vi "ISEG_HVBoard.constructor.vi"(0 "name":string, 2 "data in":string, 5 "error in (no error)":errorcluster) -> (14 "i ref out":refnum<vi>, 16 "data out":string, 19 "error out":errorcluster)   [LabVIEW 2014, in "ISEG_HVBoard.lvlib"]
doc: "This is the constructor of a class.\n\nLicense Agreement for this software:\n\nCopyright (C)\nGesellschaft für Schwerionenforschung, GSI\nPlanckstr. 1\n64291 Darmstadt\nGermany\n\nContact: D.Beck@gsi.de \n\nThis program is free software; you can redistribute it and/or modify it under the terms of the \nGNU General Public License as published by the Free Software Foundation; either version 2 of \nthe license, or (at your option) any later version.\n\nThis program is distributed in the hope that it will be useful, but WITHOUT ANY WARRANTY; \nwithout even the implied warranty of MERCHANTABILITY or FITNESS FOR A PARTICULAR PURPOSE. See the GNU General License for more details (http://www.gnu.org).\n\nGesellschaft für Schwerionenforschung, GSI\nPlanckstr. 1, 64291 Darmstadt, Germany\nFor all questions and ideas contact: M.Richter@gsi.de, H.Brand@gsi.de or D.Beck@gsi.de.\nLast update: 16-JUN-2004"
uses:
  ISEG_HVBoard.lvlib
  ISEG_HVBoard.i attribute.ctl
  ISEG_HVBoard.DIM Status.ctl
  CSCore/CSApplicationBaseClasses/DeviceBase/DeviceBase.myEventNames.ctl
  CSCore/CSApplicationBaseClasses/DeviceBase/DeviceBase.lvlib
  CSCore/CSSystem/CSSystemLib/CSSystemLib.lvlib
  CSCore/BaseProcess/BaseProcess.lvlib
panel:
  in  "CLASS.i attribute":T1 {"Status"."Status" format="%.0b"}
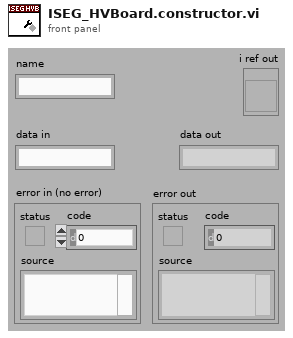
[diagram p1: front panel]
types:
  T1 = typedef "ISEG_HVBoard.lvlib/ISEG_HVBoard.i attribute.ctl" = cluster{"System Name":string, "Board ID":i32, "Prefix":string, "NrOfCh":cluster{"NrOfCh":i16, "DIM Status":T2}, "Status":cluster{"Status":i16, "DIM Status":T2}, "HardwareVLimit":cluster{"HVMax":dbl, "DIM Status":T2}, "BoardTemp":cluster{"Temp":dbl, "DIM Status":T2}, " Emcy":cluster{"Emcy":bool, "DIM Status":T2}}
  T2 = typedef "ISEG_HVBoard.lvlib/ISEG_HVBoard.DIM Status.ctl" = cluster{"no link":bool, "quality":i32, "Time Stamp":timestamp}
  T3 = enum16{"SetAttribute", "GetAttribute", "CreateAttribute", "DestroyAttribute", "DestroyAllAtributes"}
  T4 = typedef "DeviceBase.lvlib/DeviceBase.myEventNames.ctl" = enum16{"lvmsg://Initialize", "lvmsg://Close", "lvmsg://Configure", "lvmsg://Reset", "lvmsg://IDQuery"}
  T5 = typedef "BaseProcess.lvlib/BaseProcess.i attribute.ctl" = cluster{"EventStatus":string, "EventError":i32, "PresetEvtWatchD":i32, "PresetPdcWatchD":i32, "EventTimeout":i32, "PeriodicInterval":i32, "Interface":string[], "Address":string[], "Special":string[], "PeriodicError":i32, "PeriodicStatus":string, "SuperProc":string, "Descriptors":T6[], "CaseRef":refnum<vi>, "PdcRef":refnum<vi>, "Thread Ref":refnum<vi>, "eventErrorID":i32, "eventStatusID":i32, "periodicErrorID":i32, "periodicStatusID":i32, "pdcCtrID":i32}
  T6 = typedef "BaseProcess.lvlib/BaseProcess.descriptor definition.ctl" = cluster{"selector":string, "descriptor":T7}
  T7 = typedef "BaseProcess.lvlib/BaseProcess.descriptor string definition.ctl" = string
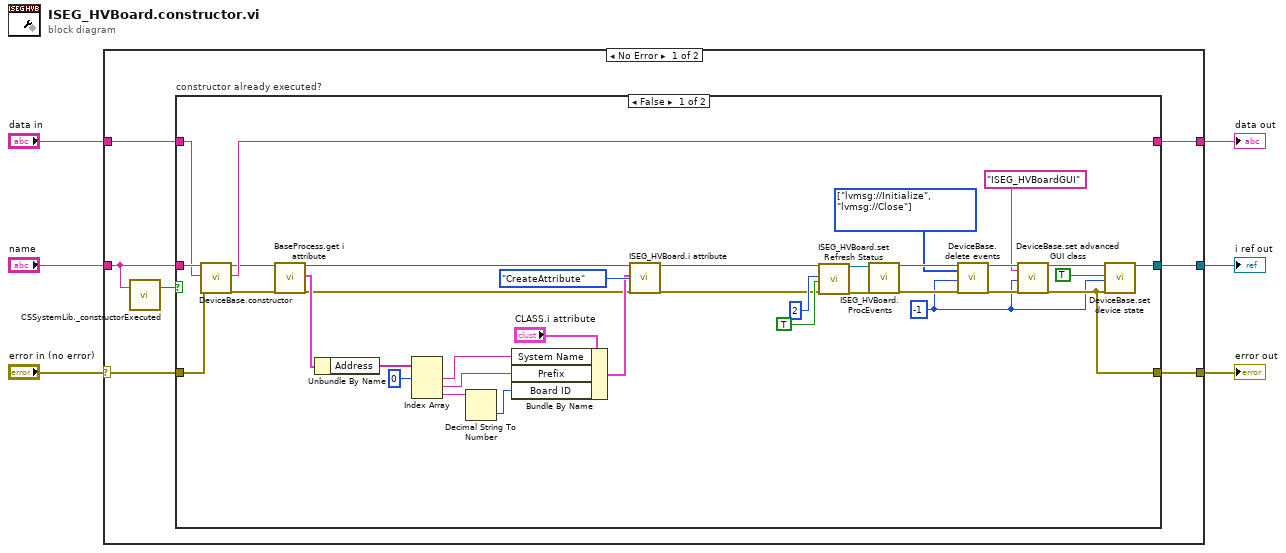
[diagram p0: block diagram]
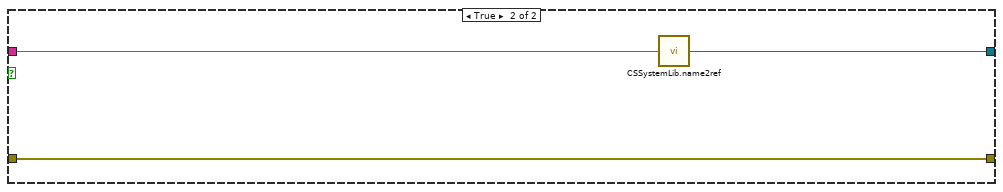
[diagram p2: hidden frame]
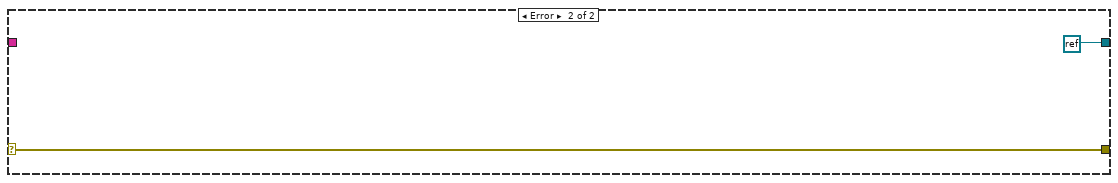
[diagram p3: hidden frame]
diagram:
  n1 = case shown="No Error" "error in (no error)" {
    selector: "error in (no error)" -> [w11 w52]
    tunnel: "name" -> [w10 _]
    tunnel: [w13 refnum<k0> refnum ("Not a Refnum Constant")] -> w5
    tunnel: [w12 w52] -> w4
    tunnel: "data in" -> [w8 _]
    tunnel: [w7 _] -> w1
    frame No Error {
      n2 = call "CSSystemLib._constructorExecuted.vi"("name"=w10) -> ("constructor executed?"=w9:bool)  [unwired: 18 in]
      n3 = case "constructor already executed?" shown="False" w9 {
        tunnel: w10 -> [w47 w51]
        tunnel: [w33 w50] -> w13
        tunnel: [w26 w49] -> w12
        tunnel: w11 -> [w46 w49]
        tunnel: w8 -> [w45 _]
        tunnel: [w41 _] -> w7
        frame False {
          w42 = T4[] [enum."lvmsg://Initialize", enum."lvmsg://Close"] items=["lvmsg://Initialize", "lvmsg://Close", "lvmsg://Configure", "lvmsg://Reset", "lvmsg://IDQuery"] ("events")
          w25 = -1 ("ms timeout (10000)")
          n4 = call "DeviceBase.constructor.vi"("name"=w47, "data in"=w45, "error in (no error)"=w46) -> ("i ref out"=w32:refnum<vi>, "data out"=w41:string, "error out"=w31:errorcluster)  [unwired: 14 in]
          n5 = call "BaseProcess.get i attribute.vi"("i ref in"=w32, "error in (no error)"=w31) -> ("i ref out"=w21:refnum<vi>, "i attribute"=w40:T5, "error out"=w20:errorcluster)  [unwired: 15 in]
          n6 = Unbundle By Name(w40) -> ("Address"=w36:string[])
          n7 = Index Array(array=w36, index #1=0 ("index")) -> (element #1=w37:string, element #2=w22:string, element #3=w23:string)  [unwired: 2 in]
          n8 = Decimal String To Number(string=w23) -> (number=w24:i32)  [unwired: 2 in, 1 out]
          n9 = Bundle By Name(cluster="CLASS.i attribute", "System Name"=w37, "Prefix"=w22, "Board ID"=w24) -> (w35:T1)
          n10 = call "ISEG_HVBoard.i attribute.vi"("VI Refnum"=w21, "CLASS.i attribute"=w35, "Action"=T3."CreateAttribute", "error in (no error)"=w20) -> ("VI Refnum out"=w15:refnum<vi>, "error out"=w14:errorcluster)  [unwired: 13 in, 1 out]
          n11 = call "ISEG_HVBoard.set Refresh Status.vi"("i ref in"=w15, "Refresh Status"=2, "Force"=TRUE, "error in (no error)"=w14) -> ("i ref out"=w16:refnum<vi>, "error out"=w17:errorcluster)  [unwired: 14 in]
          n12 = call "ISEG_HVBoard.ProcEvents.vi"("i ref in"=w16, "error in (no error)"=w17) -> ("i ref out"=w44:refnum<vi>, "error out"=w43:errorcluster)  [unwired: 16 in]
          n13 = call "DeviceBase.delete events.vi"("i ref in"=w44, "events"=w42, "ms timeout (10000)"=w25, "error in (no error)"=w43) -> ("i ref out"=w30:refnum<vi>, "error out"=w29:errorcluster)  [unwired: 13 in, 1 out]
          n14 = call "DeviceBase.set advanced GUI class.vi"("i ref in"=w30, "advancedGUIClass"="ISEG_HVBoardGUI", "ms timeout (10000)"=w25, "error in (no error)"=w29) -> ("i ref out"=w28:refnum<vi>, "error out"=w26:errorcluster)  [unwired: 13 in, 1 out]
          n15 = call "DeviceBase.set device state.vi"("i ref in"=w28, "implicit"=TRUE, "ms timeout (10000)"=w25, "error in (no error)"=w26) -> ("i ref out"=w33:refnum<vi>)  [unwired: 13 in, 2 out]
        }
        frame True {
          n16 = call "CSSystemLib.name2ref.vi"("name"=w51) -> ("obj refnum"=w50:refnum<vi>)
        }
      }
    }
    frame Error {
    }
  }
  "i ref out" <- w5
  "error out" <- w4
  "data out" <- w1
